vi "ToRepo.vi"(8 "error in":errorcluster, 9 "to repo cluster":T1, 10 "repository in":refnum<class "NISE_CEF_Repository.lvclass">, 11 "channel in":refnum<class "Channel.lvclass">) -> (0 "error out":errorcluster, 2 "repository out":refnum<class "NISE_CEF_Repository.lvclass">, 3 "channel out":refnum<class "Channel.lvclass">)   [LabVIEW 2015, in "Channel.lvclass"]
doc: "Copyright 2017 National Instruments Corporation\n\nLicensed under the Apache License, Version 2.0 (the \"License\"); you may not use this file except in compliance with the License. You may obtain a copy of the License at http://www.apache.org/licenses/LICENSE-2.0\nUnless required by applicable law or agreed to in writing, software distributed under the License is distributed on an \"AS IS\" BASIS, WITHOUT WARRANTIES OR CONDITIONS OF ANY KIND, either express or implied. See the License for the specific language governing permissions and limitations under the License."
uses:
  Channel.lvclass
  SequenceRepo/SequenceRepo.lvclass
  <vilib>/NI/Configuration Framework/Node/NISE_CEF_Node.lvclass
  <vilib>/NI/Configuration Framework/Repository/NISE_CEF_Repository.lvclass
  <vilib>/NI/Configuration Framework/Node/ToRepoCluster.ctl
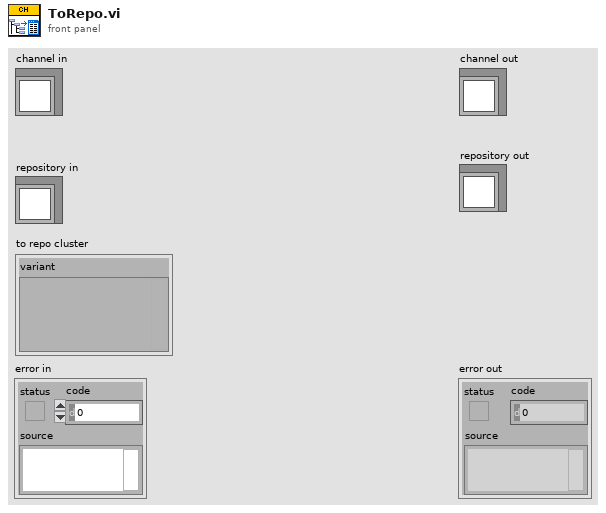
[diagram p1: front panel]
types:
  T1 = typedef "NISE_CEF_Node.lvclass/ToRepoCluster.ctl" = cluster{"variant":variant}
  T2 = typedef "Channel.ctl" = cluster{"channel group":string, "channel name":string, "IO ":string, "sensor ID":string, "description":string, "system":string, "channel type":string}
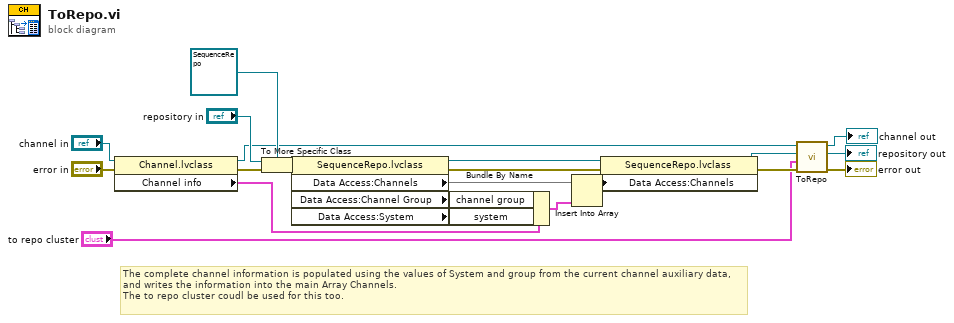
[diagram p0: block diagram]
diagram:
  # "The complete channel information is populated using the values of System and group from the current channel auxiliary data, and writes the information into the main Array Channels.\nThe to repo cluster coudl be used for this too."
  n1 = property class="Channel.lvclass"(reference="channel in", error in="error in") -> (reference out=w13:refnum<class "Channel.lvclass">, error out=w15:errorcluster, "Channel info"=w2:T2)
  n2 = To More Specific Class(target class=refnum<class "SequenceRepo.lvclass"> refnum ("cRIO repo.lvclass"), reference="repository in", error in=w15) -> (specific class reference=w18:refnum<class "SequenceRepo.lvclass">, error out=w14:errorcluster)
  n3 = property class="SequenceRepo.lvclass"(reference=w18, error in=w14) -> (reference out=w9:refnum<class "SequenceRepo.lvclass">, error out=w10:errorcluster, "Data Access:Channels"=w8, "Data Access:Channel Group"=w4, "Data Access:System"=w3)
  n4 = Bundle By Name(cluster=w2, "channel group"=w4, "system"=w3) -> (w7:T2)
  n5 = Insert Into Array(array=w8, new element=w7) -> (w6:T2[])  [unwired: 1 in]
  n6 = property class="SequenceRepo.lvclass"(reference=w9, error in=w10, "Data Access:Channels"=w6) -> (reference out=w5:refnum<class "SequenceRepo.lvclass">, error out=w11:errorcluster)
  n7 = call-parent "ToRepo.vi"("error in"=w11, "to repo cluster"="to repo cluster", "repository in"=w5, "node in"=w13) -> ("error out"=→"error out":errorcluster, "repository out"=→"repository out":refnum<class "NISE_CEF_Repository.lvclass">, "node out"=→"channel out":refnum<class "Channel.lvclass">)  [unwired: 5 in]
